vi "Calculate Plating Time DC.vi"(10 "ItemNames":string[][](array[string]), 11 "Num Steps":i32) -> (2 "Right Anode Time":dbl, 3 "Left Anode Time":dbl)   [LabVIEW 2019]
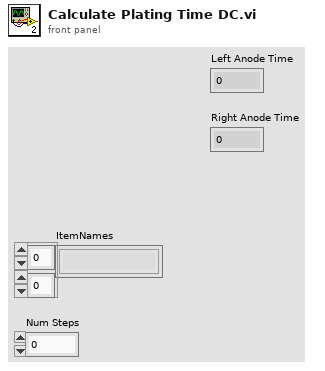
[diagram p1: front panel]
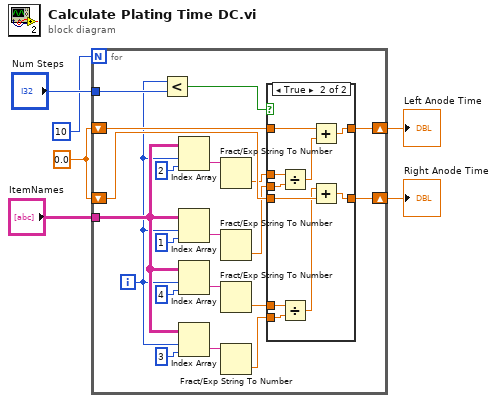
[diagram p0: block diagram]
diagram:
  w6 = 0.0 ("Numeric 3")
  n1 = for {
    N: 10 -> [_]
    tunnel: "ItemNames" -> [w12]
    tunnel: "Num Steps" -> [w24]
    shift-right: [w22] -> w1
    shift-left: w6 -> [w23]
    shift-right: [w18] -> w2
    shift-left: w6 -> [w19]
    i -> [w11]
    n2 = Less?(x=w11, y=w24) -> (x < y?=w7:bool)
    n3 = Index Array(array=w12, index (row)=w11, index (col)=2 ("disabled index (col)")) -> (element=w17:string)
    n4 = Index Array(array=w12, index (row)=w11, index (col)=1 ("disabled index (col)")) -> (element=w25:string)
    n5 = Index Array(array=w12, index (row)=w11, index (col)=4 ("disabled index (col)")) -> (element=w13:string)
    n6 = Index Array(array=w12, index (row)=w11, index (col)=3 ("disabled index (col)")) -> (element=w20:string)
    n7 = Fract/Exp String To Number(string=w17) -> (number=w15:dbl)  [unwired: 3 in, 1 out]
    n8 = Fract/Exp String To Number(string=w25) -> (number=w8:dbl)  [unwired: 3 in, 1 out]
    n9 = Fract/Exp String To Number(string=w13) -> (number=w10:dbl)  [unwired: 3 in, 1 out]
    n10 = Fract/Exp String To Number(string=w20) -> (number=w9:dbl)  [unwired: 3 in, 1 out]
    n11 = case shown="True" w7 {
      tunnel: w8 -> [_ w30]
      tunnel: w23 -> [w28 w38]
      tunnel: [w28 w37] -> w22
      tunnel: w9 -> [_ w29]
      tunnel: w19 -> [w27 w36]
      tunnel: [w27 w35] -> w18
      tunnel: w15 -> [_ w34]
      tunnel: w10 -> [_ w32]
      frame False {
      }
      frame True {
        n12 = Divide(x=w34, y=w30) -> (x/y=w33:dbl)
        n13 = Divide(x=w32, y=w29) -> (x/y=w31:dbl)
        n14 = Add(x=w38, y=w33) -> (x+y=w37:dbl)
        n15 = Add(x=w31, y=w36) -> (x+y=w35:dbl)
      }
    }
  }
  "Right Anode Time" <- w2
  "Left Anode Time" <- w1
